vi "rqp_Send Data to Debug Client.vi"(7 "Caller in":refnum<class "Worker.lvclass">, 8 "error in":errorcluster, 9 "Data in":T1, 11 "DS TCP Server in":refnum<class "DS TCP Server.lvclass">) -> (0 "error out":errorcluster, 3 "dup DS TCP Server out":refnum<class "DS TCP Server.lvclass">, 5 "dup Caller out":refnum<class "Worker.lvclass">)   [LabVIEW 2017, in "DS TCP Server.lvlib" / "DS TCP Server.lvclass"]
doc: "This VI sends a <b>Public API Request</b> message to an MHL case of the Worker that owns this VI.\n---\nForward the data to a Debug Client"
uses:
  DS TCP Server.lvclass
  C:/Program Files (x86)/National Instruments/LabVIEW 2017/vi.lib/addons/_Workers/Library/Classes/Worker/Worker.lvclass
  <vilib>/addons/_Workers/Library/Classes/Worker/Worker.lvclass
  rqp_Send Data to Debug Client.ctl
  Common VIs/DC_UID.ctl
  <vilib>/addons/_Workers/Library/Classes/Worker/Worker.lvclass/Worker.ctl
  <vilib>/addons/_Workers/Library/Classes/Message/Priority.ctl
  <vilib>/addons/_Workers/Library/Classes/Message/Enqueue Message to Queue.vi
  <vilib>/addons/_Workers/Library/Classes/Message/Message.lvclass
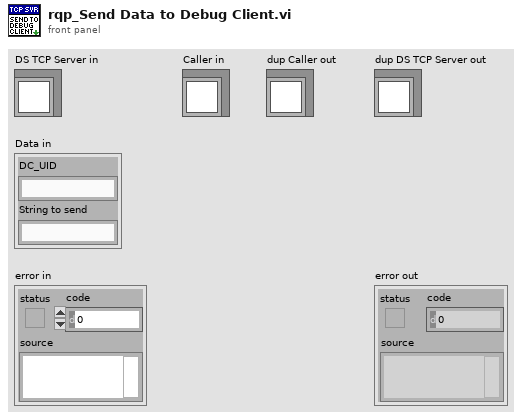
[diagram p1: front panel]
types:
  T1 = typedef "DS TCP Server.lvlib/DS TCP Server.lvclass/rqp_Send Data to Debug Client.ctl" = cluster{"DC_UID":T2, "String to send":string}
  T2 = typedef "DC_UID.ctl" = string
  T3 = typedef "Workers.lvlib/Message.lvclass/Priority.ctl" = enum16{"Low", "Normal", "High"}
  T4 = typedef "Workers.lvlib/Case Label.ctl" = string
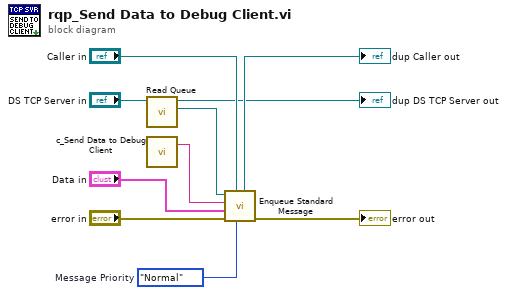
[diagram p0: block diagram]
diagram:
  w6 = Priority."Normal"  # Message Priority
  n1 = call <vilib>:"Read Queue.vi"("Worker_"="DS TCP Server in") -> ("Message Queue out"=w2:refnum<class "Message Queue.lvclass">, "dup Worker_out"=→"dup DS TCP Server out":refnum<class "DS TCP Server.lvclass">)  [unwired: 9 in]
  n2 = call "c_Send Data to Debug Client.vi"() -> ("Case Label"=w5:T4)  [unwired: 1 in]
  n3 = call-poly <vilib>:"Enqueue Standard Message.vi"("Priority (Normal)"=w6, "Worker"="Caller in", "error in"="error in", "Data"="Data in", "Case Label"=w5, "Message Queue"=w2) -> ("error out"=→"error out":errorcluster, "dup Worker out"=→"dup Caller out":refnum<class "Worker.lvclass">)  [unwired: 3 in, 1 out]
